vi "setCameraEventsManger.vi"(8 "error in (no error)":errorcluster, 10 "Hardware:Channels.lvlib:CameraEventsManger.lvclass":refnum<class "CameraEventsManger.lvclass">, 11 "CameraController.lvclass in":refnum<class "CameraController.lvclass">) -> (0 "error out":errorcluster, 3 "CameraController.lvclass out":refnum<class "CameraController.lvclass">)   [LabVIEW 2011, in "Hardware.lvlib" / "Channels.lvlib" / "CameraController.lvclass"]
uses:
  CameraController.lvclass
  CameraEventsManager/CameraEventsManger.lvclass
  CameraController.lvclass/CameraController.ctl
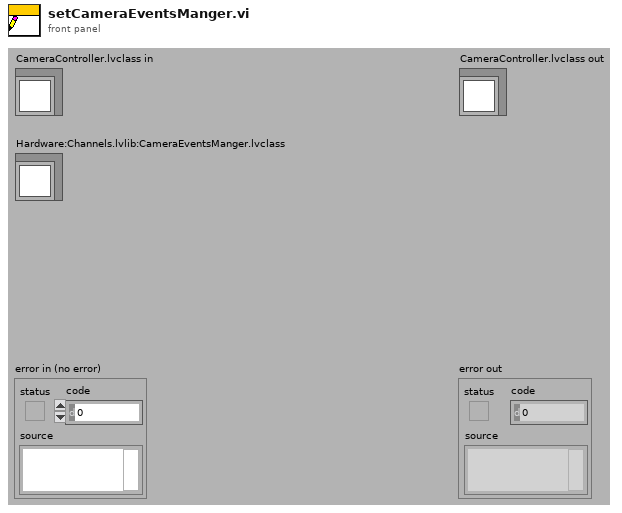
[diagram p1: front panel]
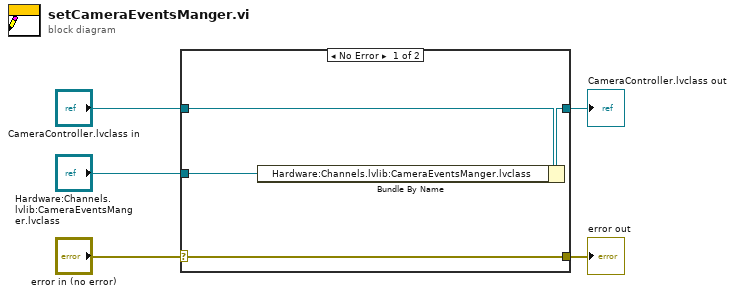
[diagram p0: block diagram]
diagram:
  n1 = case shown="No Error" "error in (no error)" {
    selector: "error in (no error)" -> [w9 w10]
    tunnel: [w9 w10] -> w4
    tunnel: [w7 w11] -> w2
    tunnel: "CameraController.lvclass in" -> [w8 w11]
    tunnel: "Hardware:Channels.lvlib:CameraEventsManger.lvclass" -> [w6 _]
    frame No Error {
      n2 = Bundle By Name(cluster=w8, "Hardware:Channels.lvlib:CameraEventsManger.lvclass"=w6) -> (w7:refnum<class "CameraController.lvclass">)
    }
    frame Error {
    }
  }
  "error out" <- w4
  "CameraController.lvclass out" <- w2
